vi "DIRECT_RATING_PRINT.vi"(7 "PRN Data":string="^XA\n^CF0,30\n^FO50,50^FD%S3A %S1 CURVE^FS\n^FO70,100^FD%S4mA %S2^FS\n^XZ\n", 8 "error in":errorcluster, 11 "Printer IP":string) -> (0 "error out":errorcluster)   [LabVIEW 2017]
uses:
  58bdaf06-725e-4811-b1ec-4c089fbf3de4.vi
  db34f251-0fed-4f13-9e22-50a6bf039d06.vi
  Global/PLC_to_Auto.vi
panel:
  out "Array":string[](array[string])
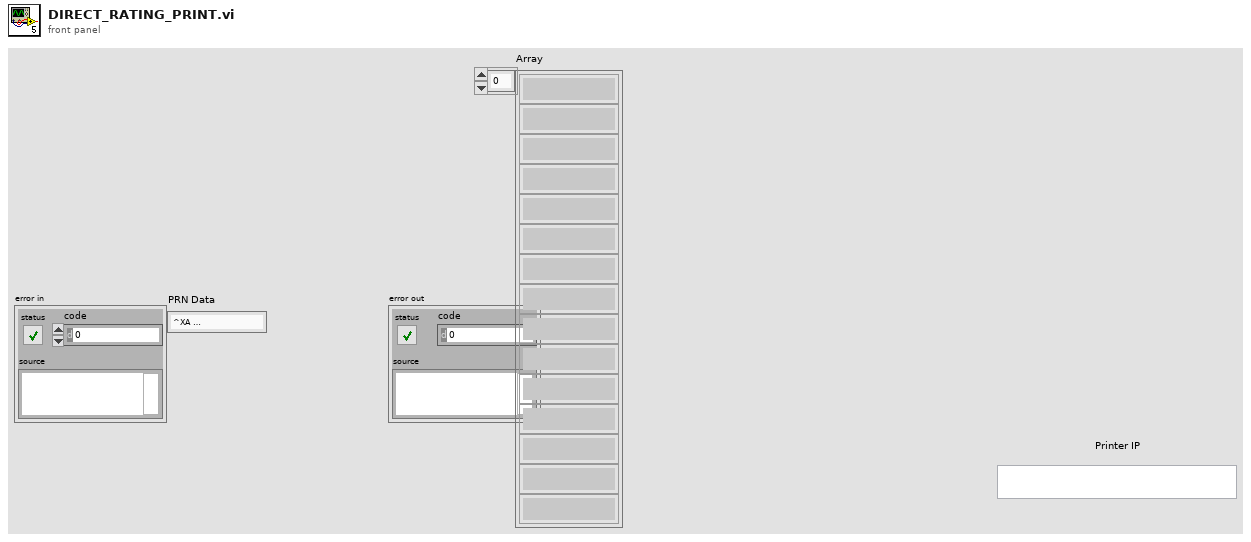
[diagram p1: front panel]
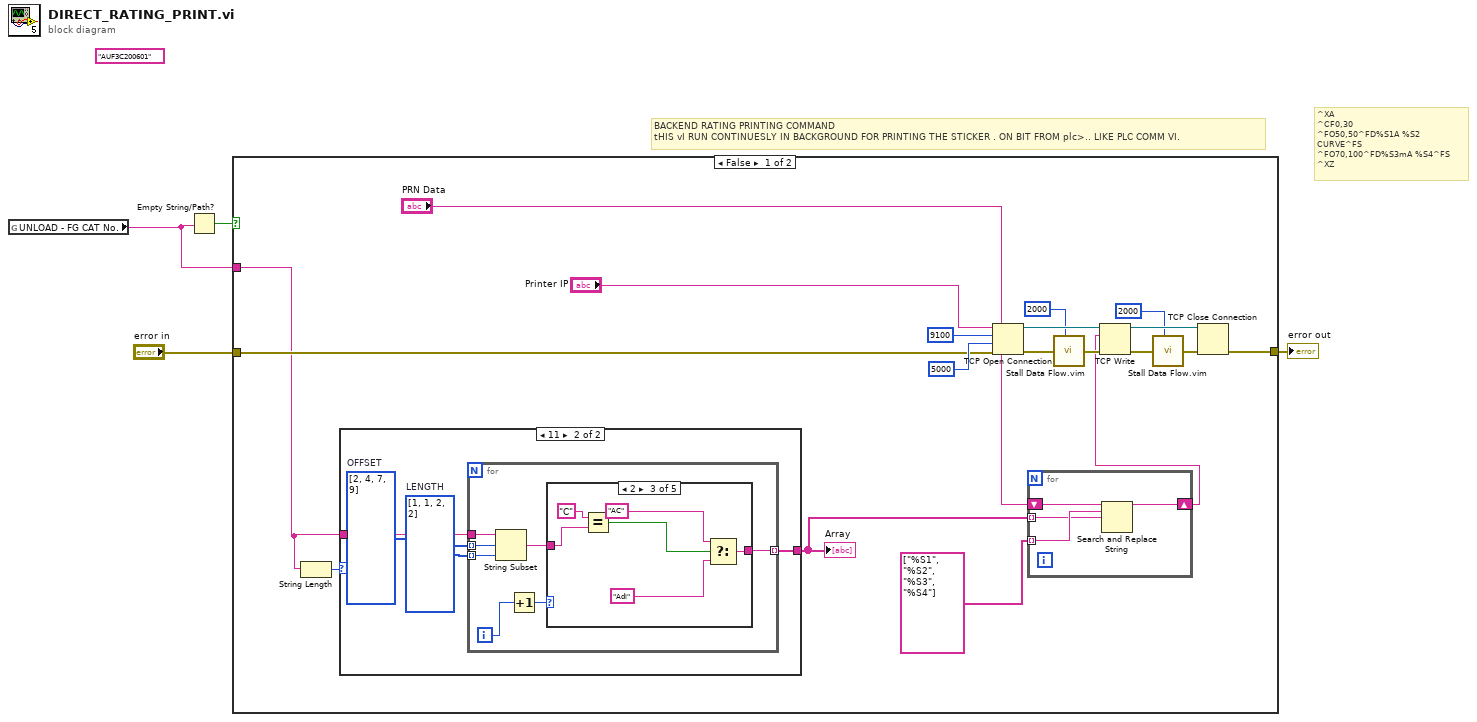
[diagram p0: block diagram]
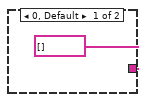
[diagram p2: hidden frame]
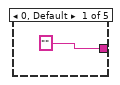
[diagram p3: hidden frame]
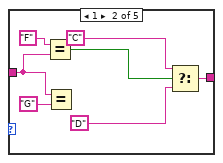
[diagram p4: hidden frame]
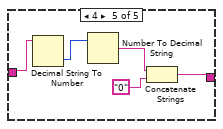
[diagram p6: hidden frame]
diagram:
  (unwired) "AUF3C200601"
  # "^XA\n^CF0,30\n^FO50,50^FD%S1A %S2 CURVE^FS\n^FO70,100^FD%S3mA %S4^FS\n^XZ"
  # "BACKEND RATING PRINTING COMMAND\ntHIS vI RUN CONTINUESLY IN BACKGROUND FOR PRINTING THE STICKER . ON BIT FROM plc>.. LIKE PLC COMM VI."
  n1 = global read "PLC_to_Auto.vi" "UNLOAD - FG CAT No."() -> (w1:string)
  n2 = Empty String/Path?(string/path=w1) -> (empty?=w4:bool)
  n3 = case shown="False" w4 {
    tunnel: w1 -> [w7 _]
    tunnel: [w13 w60] -> w3
    tunnel: "error in" -> [w12 w60]
    frame False {
      n4 = String Length(string=w7) -> (length=w10:i32)
      n5 = case shown="11" w10 {
        tunnel: w7 -> [_ w28]
        tunnel: [string[] [] w25] -> w8
        frame 0, Default {
        }
        frame 11 {
          w27 = i32[] [2, 4, 7, 9]  # OFFSET
          w26 = i32[] [1, 1, 2, 2]  # LENGTH
          n6 = for {
            tunnel: w28 -> [w35]
            tunnel: w27 -> [w34] mode=indexing
            tunnel: w26 -> [w33] mode=indexing
            tunnel: [w29] -> w25 mode=indexing
            i -> [w32]
            n7 = String Subset(string=w35, offset (0)=w34, length (rest)=w33) -> (substring=w31:string)
            n8 = Increment(x=w32) -> (x+1=w30:i32)
            n9 = case shown="2" w30 {
              tunnel: w31 -> [_ w43 w49 w50 w52]
              tunnel: ["" w37 w44 w50 w55] -> w29
              frame 0, Default {
              }
              frame 1 {
                n10 = Equal?(x="F", y=w43) -> (x = y?=w40:bool)
                n11 = Equal?(x=w43, y="G") -> ()  [unwired: 1 out]
                n12 = Select(t="C", s=w40, f="D") -> (s? t:f=w37:string)
              }
              frame 2 {
                n13 = Equal?(x="C", y=w49) -> (x = y?=w47:bool)
                n14 = Select(t="AC", s=w47, f="Adi") -> (s? t:f=w44:string)
              }
              frame 3 {
              }
              frame 4 {
                n15 = Decimal String To Number(string=w52) -> (number=w53:i32)  [unwired: 2 in, 1 out]
                n16 = Number To Decimal String(number=w53) -> (decimal integer string=w51:string)  [unwired: 1 in]
                n17 = Concatenate Strings(w51, "0") -> (w55:string)
              }
            }
          }
        }
      }
      "Array" <- w8
      n18 = TCP Open Connection(address="Printer IP", remote port or service name=9100 ("timeout ms (60000)"), timeout ms (60000)=5000, error in (no error)=w12) -> (connection ID=w22:refnum<k5>, error out=w21:errorcluster)  [unwired: 1 in]
      n19 = for {
        tunnel: string[] ["%S1", "%S2", "%S3", "%S4"] -> [w58] mode=indexing
        shift-right: [w57] -> w6
        shift-left: "PRN Data" -> [w59]
        tunnel: w8 -> [w56] mode=indexing
        n20 = Search and Replace String(input string=w59, search string=w58, replace string=w56) -> (result string=w57:string)  [unwired: 5 in, 3 out]
      }
      n21 = call "Stall Data Flow.vim"("value in"=w21, "milliseconds to wait"=u32 2000) -> ("value out"=w19:errorcluster)  [unwired: 1 out]
      n22 = TCP Write(connection ID=w22, data in=w6, error in (no error)=w19) -> (connection ID out=w20:refnum<k5>, error out=w23:errorcluster)  [unwired: 2 out]
      n23 = call "Stall Data Flow.vim"("value in"=w23, "milliseconds to wait"=u32 2000) -> ("value out"=w18:errorcluster)  [unwired: 1 out]
      n24 = TCP Close Connection(connection ID=w20, error in (no error)=w18) -> (error out=w13:errorcluster)  [unwired: 2 out]
    }
    frame True {
    }
  }
  "error out" <- w3
